vi "GCMPlugin_IsSupportingItem.vi"(8 "error in (no error)":errorcluster, 9 "VI Reference":refnum<vi>, 10 "ProjectItem Refnum":refnum<vi>, 11 "_Default in":refnum<class "FPGAChannelsManager.lvclass">) -> (0 "error out":errorcluster, 2 "IsSupportingItem":bool, 3 "_Default out":refnum<class "FPGAChannelsManager.lvclass">)   [LabVIEW 2015, in "FPGAChannelsManager.lvclass"]
uses:
  FPGAChannelsManager.lvclass
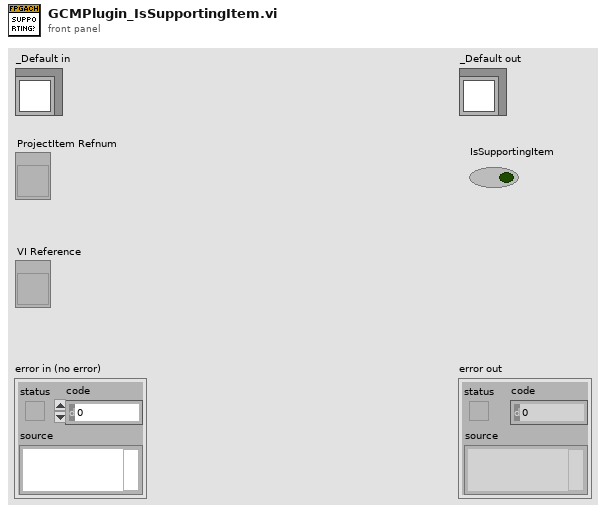
[diagram p1: front panel]
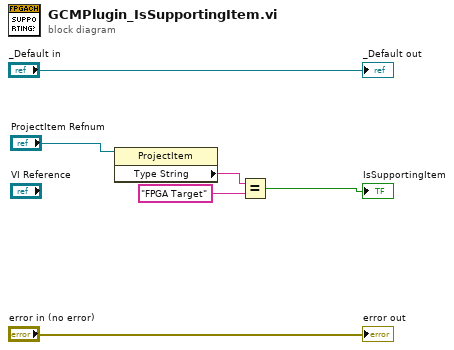
[diagram p0: block diagram]
diagram:
  n1 = property class="ProjectItem"(reference="ProjectItem Refnum") -> ("Type String"=w3:string)  [unwired: 1 in, 2 out]
  n2 = Equal?(x=w3, y="FPGA Target") -> (x = y?=→"IsSupportingItem":bool)
  "error out" <- "error in (no error)"
  "_Default out" <- "_Default in"
